vi "Init.vi"(8 "error in (no error)":errorcluster, 11 "Path":path) -> (0 "error out":errorcluster, 3 "Config-JSON out":refnum<class "Config-JSON.lvclass">)   [LabVIEW 2020, in "CDM-Config.lvlib" / "Config-JSON.lvclass"]
uses:
  Config-JSON.lvclass
  Config-JSON.lvclass/Config-JSON.ctl
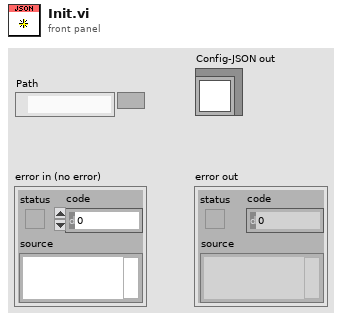
[diagram p1: front panel]
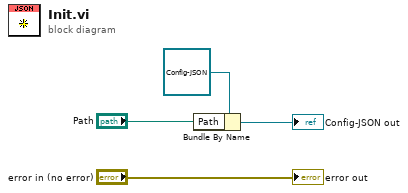
[diagram p0: block diagram]
diagram:
  n1 = Bundle By Name(cluster=refnum<class "Config-JSON.lvclass"> refnum ("Config-JSON in"), "Path"="Path") -> (→"Config-JSON out":refnum<class "Config-JSON.lvclass">)
  "error out" <- "error in (no error)"
